vi "To And From String Array Test.vi"() -> ()   [LabVIEW 2015, in "StepTests.lvlib"]
uses:
  StepTests.lvlib
  Config/Step Config.lvclass
panel:
  out "error out":errorcluster
  out "Pass":bool
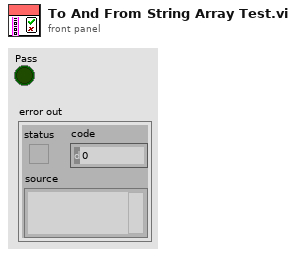
[diagram p1: front panel]
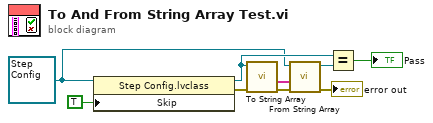
[diagram p0: block diagram]
diagram:
  w1 = refnum<class "Step Config.lvclass"> refnum ("Step Config.lvclass")
  n1 = property class="Step Config.lvclass"(reference=w1, "Skip"=TRUE) -> (reference out=w5:refnum<class "Step Config.lvclass">, error out=w2:errorcluster)  [unwired: 1 in]
  n2 = call-dynamic "To String Array.vi"("error in (no error)"=w2, "Step Config in"=w5) -> ("error out"=w8:errorcluster, "Step String Array"=w9:string[])  [unwired: 7 in, 1 out]
  n3 = call-dynamic "From String Array.vi"("error in (no error)"=w8, "String Array"=w9, "Step Config in"=w1) -> ("error out"=→"error out":errorcluster, "Step Config out"=w6:refnum<class "Step Config.lvclass">)  [unwired: 7 in]
  n4 = Equal?(x=w5, y=w6) -> (x = y?=→"Pass":bool)
